vi "1Cx2x3-Small RC.vi"   [LabVIEW 2011]
panel:
  # "this is the parent VI under which the Small RC Boat's sensors, RIO and OCU run.\nUNDER DEVELOPMENT by Jason"
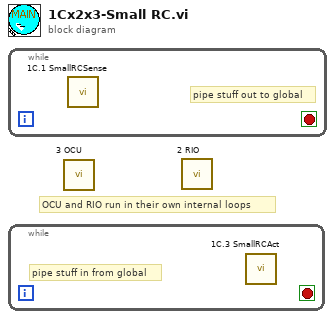
[diagram p0: block diagram]
diagram:
  # "OCU and RIO run in their own internal loops"
  n1 = while {
    stop <- _ stop-if-true
    # "pipe stuff out to global"
    n2 = call "1C.1 SmallRCSense.vi"() -> ()  [unwired: 12 in]
  }
  n3 = while {
    stop <- _ stop-if-true
    # "pipe stuff in from global"
    n4 = call "1C.3 SmallRCAct.vi"() -> ()  [unwired: 12 in]
  }
  n5 = call "3 OCU.vi"() -> ()  [unwired: 12 in]
  n6 = call "2 RIO.vi"() -> ()  [unwired: 12 in]
